vi "Configure Serial Bus (Chart Serial Signal).vi"(0 "VISA resource name":refnum<visa-resource-name>, 1 "Mode (1: Roll)":i32(ring)=1 items=["Main", "Roll"], 5 "Math Function Number (1)":i32=1, 7 "Offset (-0.25)":dbl=-0.25, 9 "Chart Signal Source (0: SBUS1)":i32(ring) items=["SBUS1", "SBUS2"], 11 "error in (no error)":errorcluster, 12 "Time Range (0.5)":dbl=0.5) -> (4 "VISA resource name out":refnum<visa-resource-name>, 15 "error out":errorcluster)   [LabVIEW 2015, in "Agilent 2000 3000 X-Series.lvlib"]
doc: "Configures chart serial signal"
uses:
  Agilent 2000 3000 X-Series.lvlib
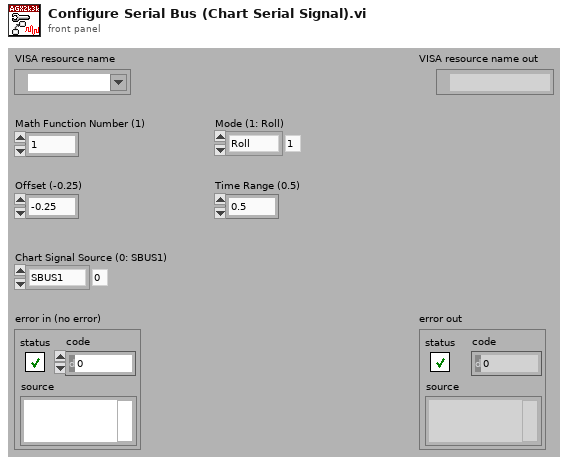
[diagram p1: front panel]
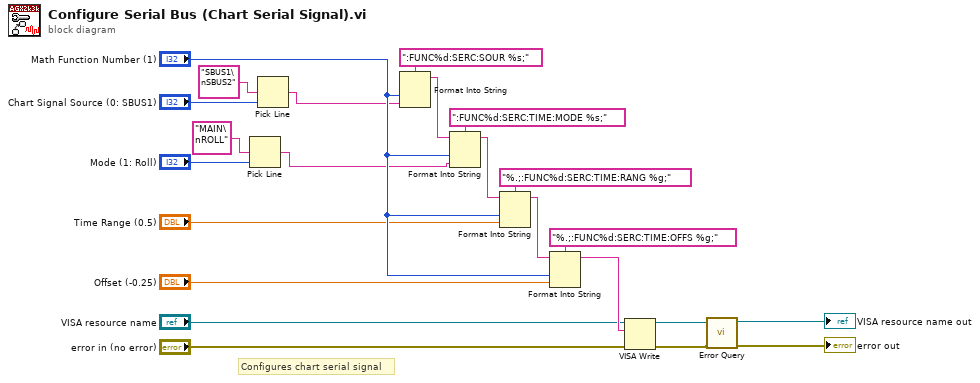
[diagram p0: block diagram]
diagram:
  # "Configures chart serial signal"
  n1 = Pick Line(multi-line string="MAIN\nROLL", line index="Mode (1: Roll)") -> (output string=w4:string)  [unwired: 1 in]
  n2 = Pick Line(multi-line string="SBUS1\nSBUS2", line index="Chart Signal Source (0: SBUS1)") -> (output string=w1:string)  [unwired: 1 in]
  n3 = Format Into String(format string=":FUNC%d:SERC:SOUR %s;", "Math Function Number (1)", w1) -> (resulting string=w21:string)  [unwired: 2 in, 1 out]
  n4 = Format Into String(format string=":FUNC%d:SERC:TIME:MODE %s;", initial string=w21, "Math Function Number (1)", w4) -> (resulting string=w19:string)  [unwired: 1 in, 1 out]
  n5 = Format Into String(format string="%.;:FUNC%d:SERC:TIME:RANG %g;", initial string=w19, "Math Function Number (1)", "Time Range (0.5)") -> (resulting string=w16:string)  [unwired: 1 in, 1 out]
  n6 = Format Into String(format string="%.;:FUNC%d:SERC:TIME:OFFS %g;", initial string=w16, "Math Function Number (1)", "Offset (-0.25)") -> (resulting string=w13:string)  [unwired: 1 in, 1 out]
  n7 = VISA Write(VISA resource name="VISA resource name", write buffer=w13, error in (no error)="error in (no error)") -> (VISA resource name out=w10:refnum<visa-resource-name>, error out=w9:errorcluster)  [unwired: 1 out]
  n8 = call "Error Query.vi"("error in (no error)"=w9, "VISA resource name"=w10) -> ("error out"=→"error out":errorcluster, "VISA resource name out"=→"VISA resource name out":refnum<visa-resource-name>)  [unwired: 6 in, 2 out]
